vi "statetransit.vi"() -> ()   [LabVIEW 2020]
uses:
  <extravilib>/ChannelInstances/Tag-u16[State 1,State 2,State 3].lvlib
  <extravilib>/ChannelInstances/Tag-bool.lvlib
panel:
  out "Current State 1":enum16{"State 1", "State 2", "State 3"}(ring)
  out "State 1 Indicator":bool
  out "State 2 Indicator":bool
  out "Current State 2":enum16{"State 1", "State 2", "State 3"}(ring)
  in  "StateEnum Def":enum16{"State 1", "State 2", "State 3"}(ring)
  out "Current State":enum16{"State 1", "State 2", "State 3"}(ring)
  in  "Stop":bool
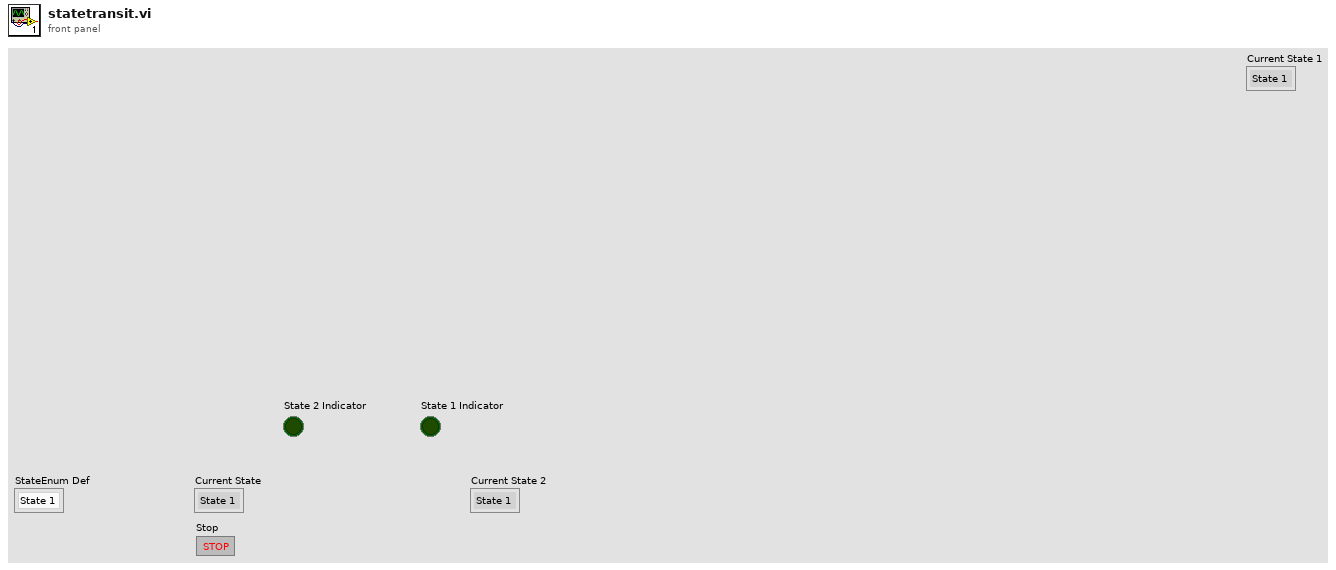
[diagram p1: front panel]
types:
  T1 = typedef "Tag-u16[State 1,State 2,State 3].lvlib/))Channel.ctl" = refnum<queue>
  T2 = typedef "Tag-bool.lvlib/))Channel.ctl" = refnum<queue>
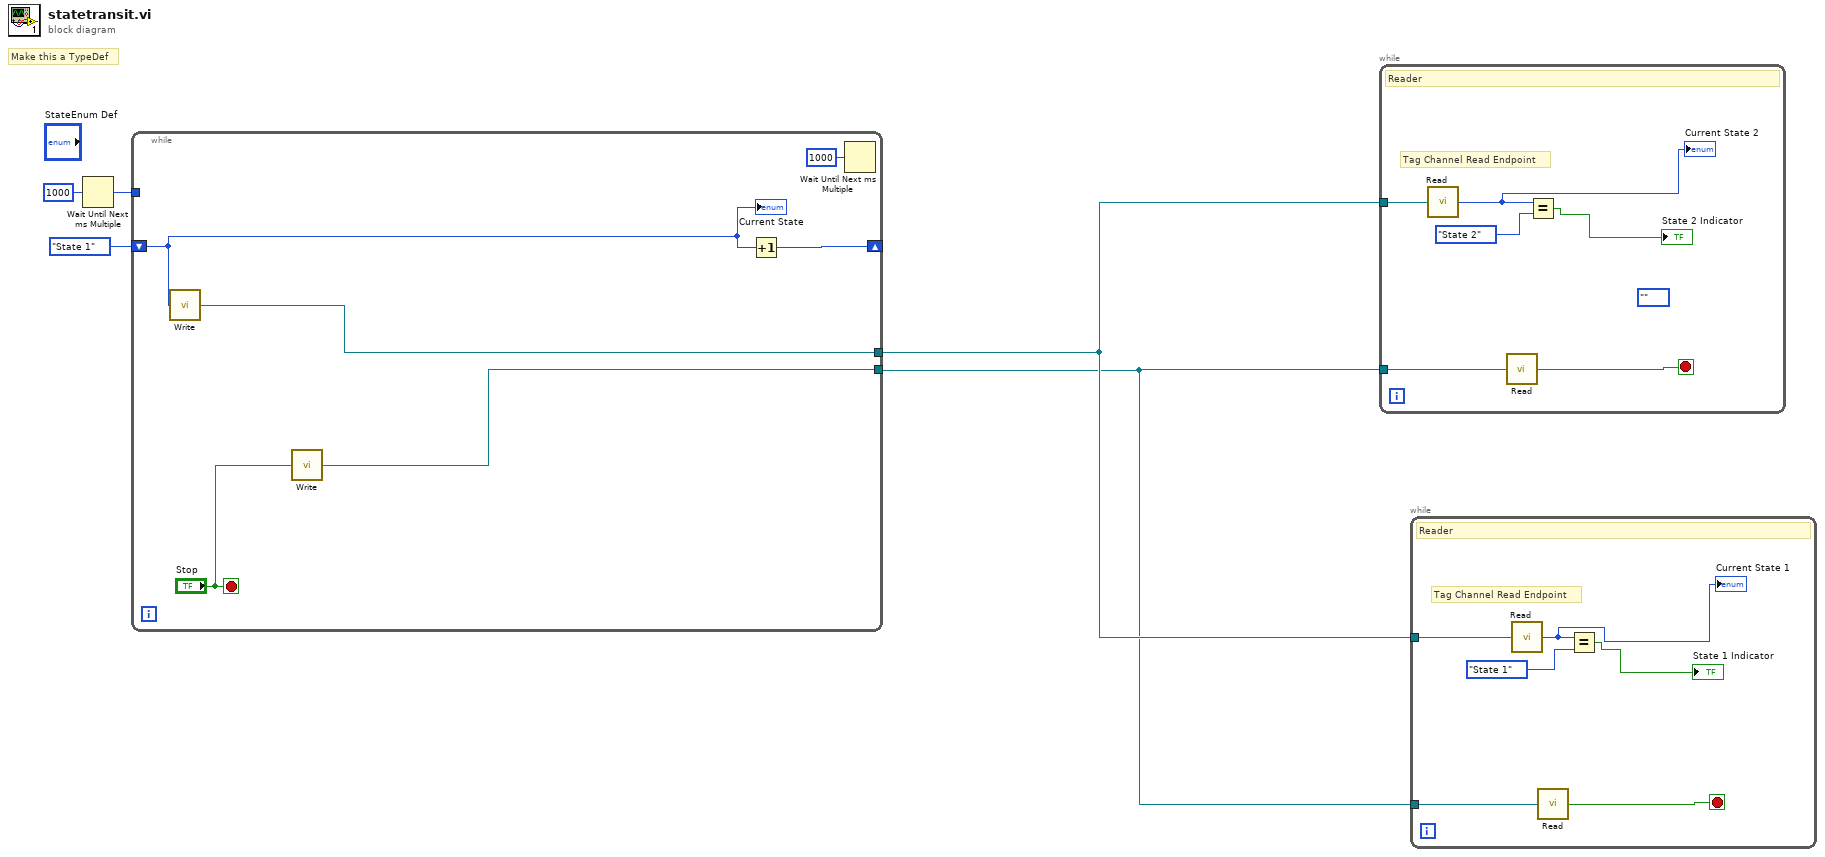
[diagram p0: block diagram]
diagram:
  # "Make this a TypeDef"
  n1 = Wait Until Next ms Multiple(millisecond multiple=u32 1000) -> (millisecond timer value=w3:u32)
  n2 = while {
    shift-right: [w10] -> _
    shift-left: enum16{"State 1", "State 2", "State 3"}."State 1" ("Current State") -> [w9]
    tunnel: w3 -> [_]
    tunnel: [w8] -> w2
    tunnel: [w6] -> w1
    stop <- "Stop" stop-if-true
    n3 = call <extravilib>:"Write.vi"("element"=w9) -> ("channel"=w8:T1)  [unwired: 1 out]
    n4 = call <extravilib>:"Write.vi"("element"="Stop") -> ("channel"=w6:T2)  [unwired: 1 out]
    n5 = Increment(x=w9) -> (x+1=w10:enum16{"State 1", "State 2", "State 3"})
    n6 = Wait Until Next ms Multiple(millisecond multiple=u32 1000) -> ()  [unwired: 1 out]
    "Current State" <- w9
  }
  n7 = while {
    tunnel: w2 -> [w15]
    tunnel: w1 -> [w17]
    stop <- w16 stop-if-true
    (unwired) enum16{""}.""
    # "Tag Channel Read Endpoint"
    # "Reader"
    n8 = call <extravilib>:"Read.vi"("channel"=w15) -> ("element"=w12:enum16{"State 1", "State 2", "State 3"})  [unwired: 1 in, 1 out]
    "Current State 2" <- w12
    n9 = call <extravilib>:"Read.vi"("channel"=w17) -> ("element"=w16:bool)  [unwired: 1 in, 1 out]
    n10 = Equal?(x=w12, y=enum16{"State 2"}."State 2") -> (x = y?=→"State 2 Indicator":bool)
  }
  n11 = while {
    tunnel: w2 -> [w21]
    tunnel: w1 -> [w23]
    stop <- w22 stop-if-true
    # "Tag Channel Read Endpoint"
    # "Reader"
    n12 = call <extravilib>:"Read.vi"("channel"=w21) -> ("element"=w18:enum16{"State 1", "State 2", "State 3"})  [unwired: 1 in, 1 out]
    "Current State 1" <- w18
    n13 = call <extravilib>:"Read.vi"("channel"=w23) -> ("element"=w22:bool)  [unwired: 1 in, 1 out]
    n14 = Equal?(x=w18, y=enum16{"State 1"}."State 1") -> (x = y?=→"State 1 Indicator":bool)
  }
